vi "File IO.vi"() -> ()   [LabVIEW 2018]
uses:
  <vilib>/Utility/sysdir.llb/System Directory Type.ctl
  <vilib>/Utility/file.llb/Write Delimited Spreadsheet (DBL).vi
  <vilib>/Utility/file.llb/Write Delimited Spreadsheet (string).vi
panel:
  out "Waveform Chart":dbl[](graph)
  in  "Disabled":T1(ring)
  in  "Slide 2":dbl(slide) scale=-100.0..100.0
  in  "Slide":dbl(slide) scale=-100.0..100.0
  in  "Boolean":bool
  in  "Send":bool
  in  "stop":bool
  in  "Cluster":T2
  in  "count":i32
  out "error out 3":errorcluster
  out "text 2":string
  out "error out 2":errorcluster
  in  "text":string
  out "error out":errorcluster
  out "appended path":path
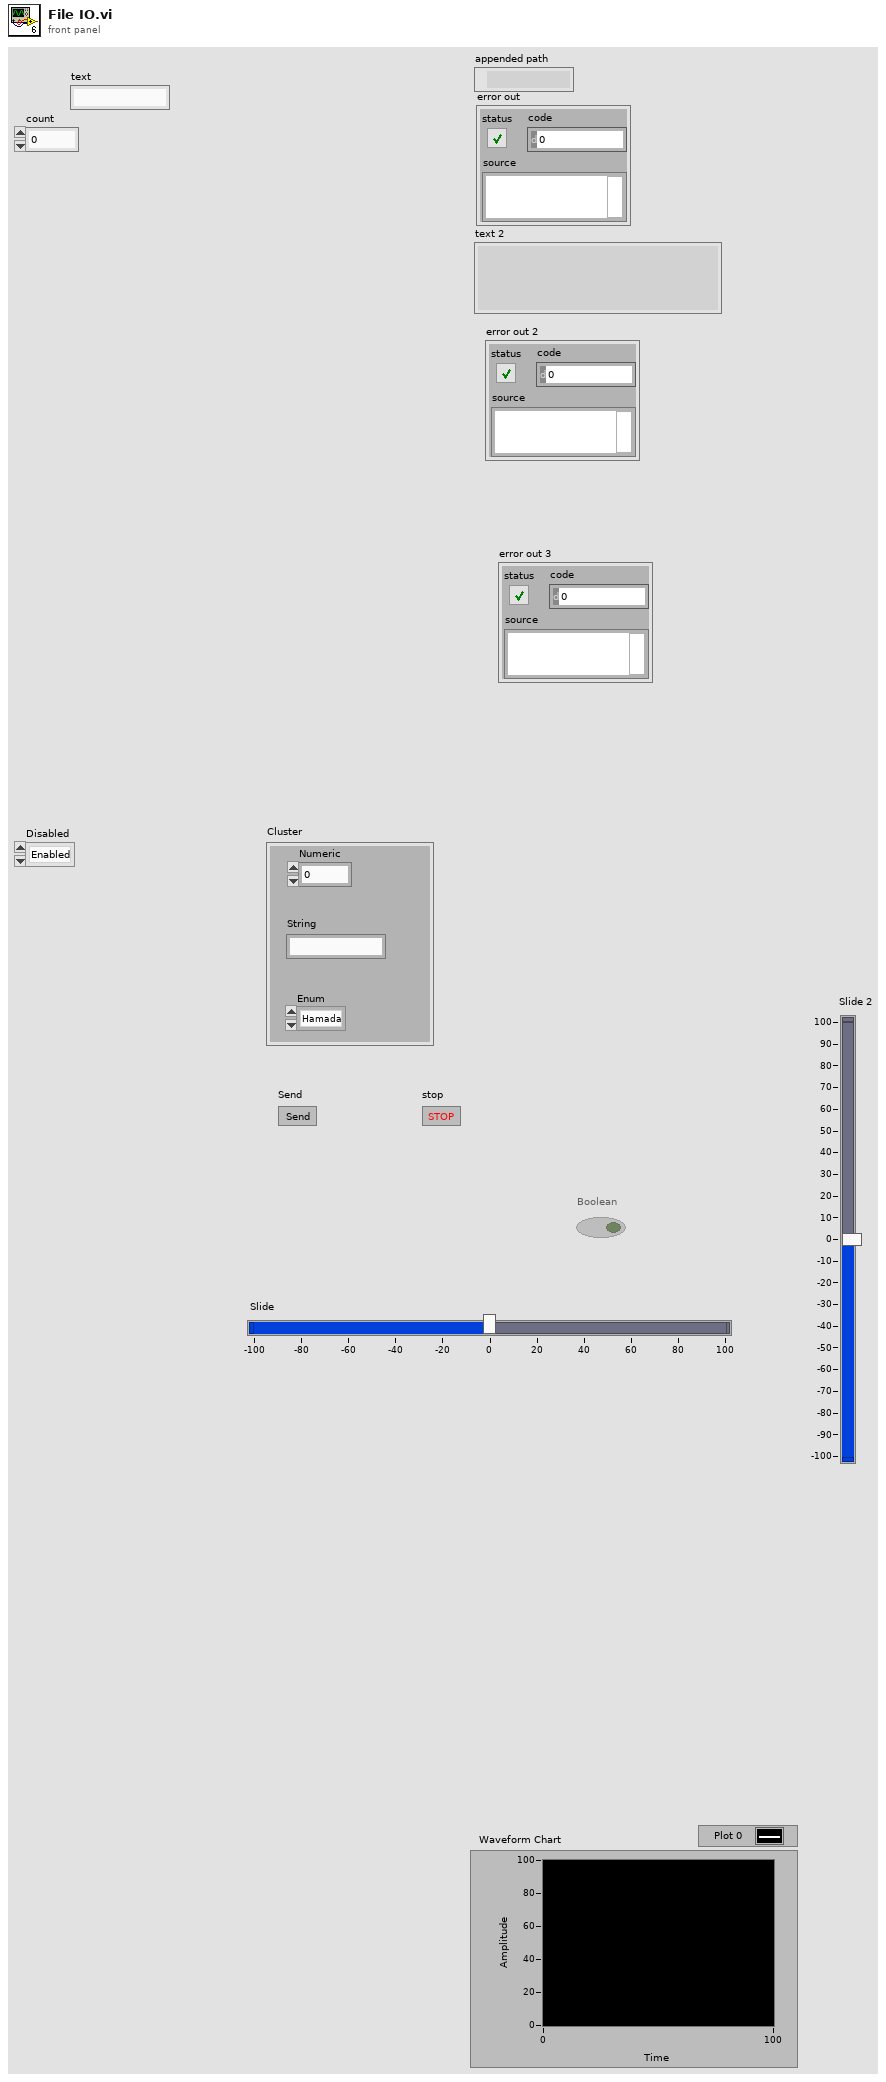
[diagram p1: front panel]
types:
  T1 = enum8{"Enabled", "Disabled", "Disabled and Grayed Out"}
  T2 = cluster{"Numeric":dbl, "String":string, "Enum":enum16{"Hamada"}}
  T3 = typedef "System Directory Type.ctl" = i32
  T4 = enum16{"open", "replace", "create", "open or create", "replace or create", "replace or create with confirmation"}
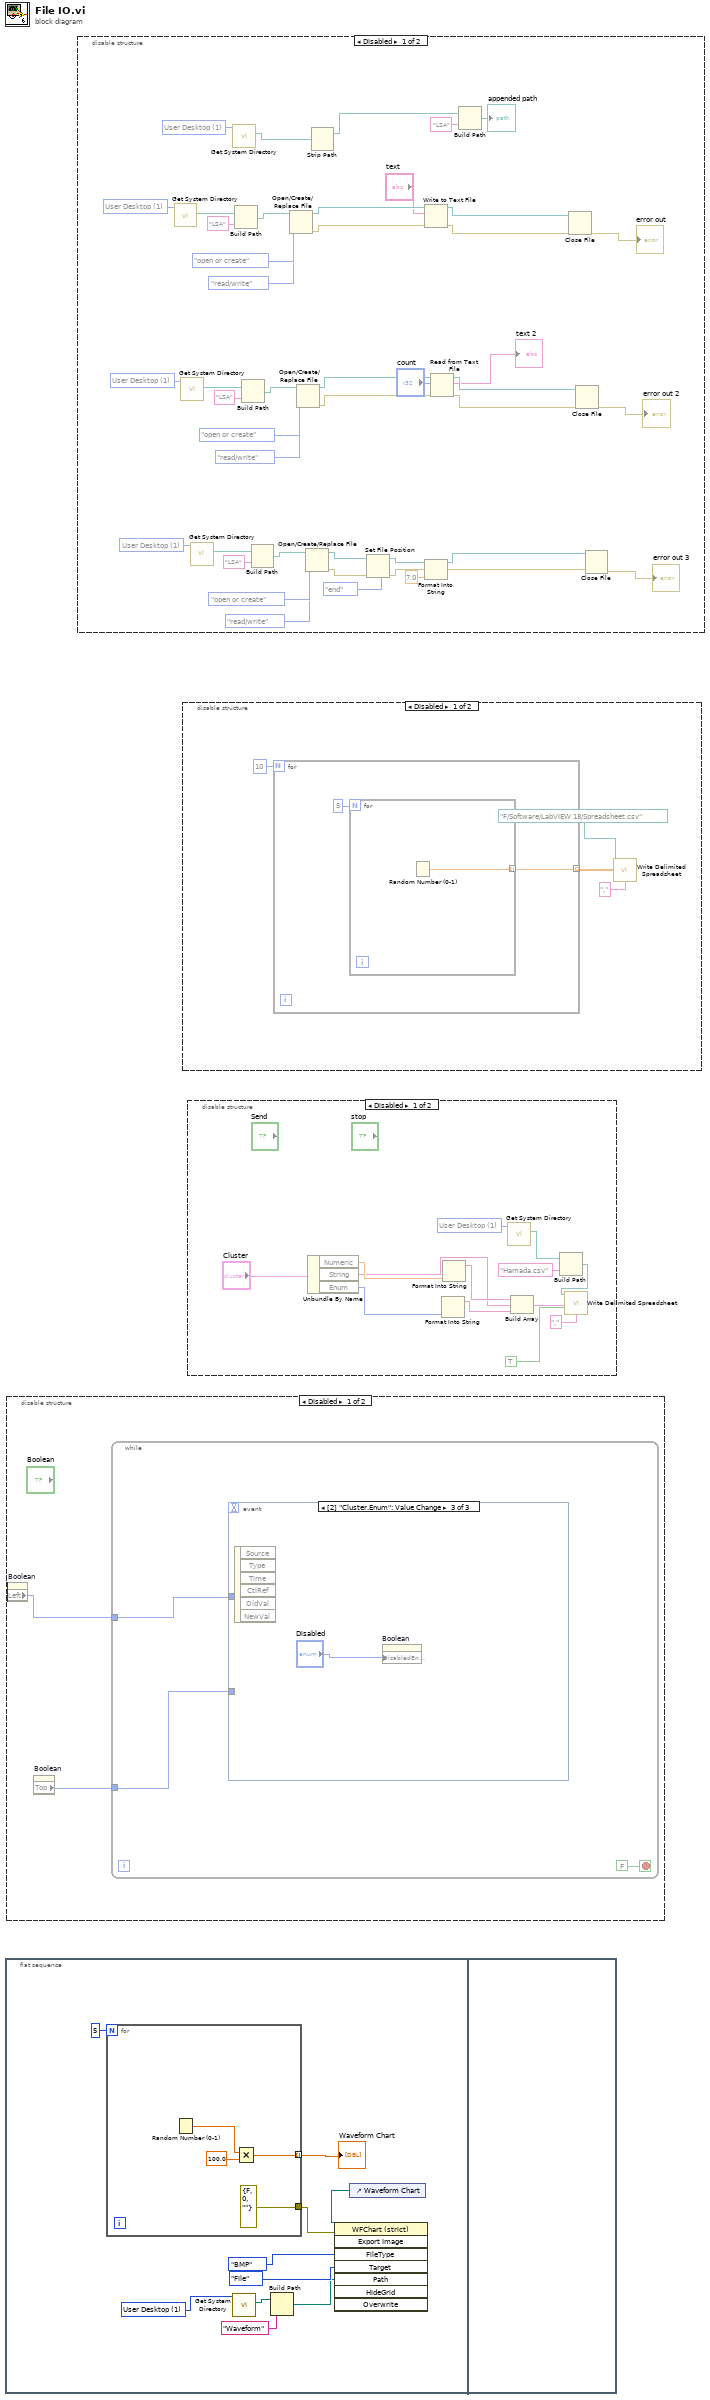
[diagram p0: block diagram]
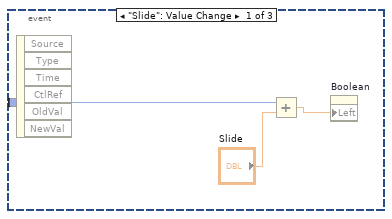
[diagram p2: hidden frame]
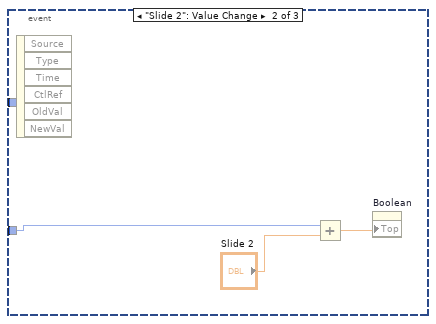
[diagram p3: hidden frame]
diagram:
  n1 = flat-sequence {
    frame #0 {
      w2 = T3 1 items=["User Home"=0, "User Desktop"=1, "User Documents"=2, "User Application Data"=3, "User Preferences"=4, "User Temporary"=5, "Public Documents"=6, "Public Application Data"=7, "Public Preferences"=8, "Public Cache"=13, "System Core Libraries"=9, "System Installed Libraries"=10, "Application Files"=11, "Boot Volume Root"=12] ("system directory type")
      n2 = for {
        N: 5 -> [_]
        tunnel: [w12] -> w9 mode=indexing
        tunnel: [errorcluster {"status"=FALSE, "code"=0, "source"=""} ("error in (no error)")] -> w7
        n3 = Random Number (0-1)() -> (number: 0 to 1=w14:dbl)
        n4 = Multiply(x=w14, y=100.0) -> (x*y=w12:dbl)
      }
      "Waveform Chart" <- w9
      n5 = call <vilib>:"Get System Directory.vi"("system directory type"=w2) -> ("system directory"=w3:path)  [unwired: 10 in]
      n6 = Build Path(base path=w3, name or relative path="Waveform") -> (appended path=w1:path)
      n7 = control-ref of="Waveform Chart"() -> (w8:refnum<vi>)
      n8 = invoke class="WFChart (strict)" method="Export Image"(reference=w8, error in=w7, "FileType"=enum32{"BMP", "EPS", "EMF", "PICT"}."BMP" ("File Type"), "Target"=enum32{"File", "Clipboard"}."File", "Path"=w1) -> ()  [unwired: 3 in, 8 out]
    }
    frame #1 {
    }
  }
  n9 = disable-structure shown="Disabled" {
    frame Disabled {
      n10 = property on="Boolean" class="Bool (strict)"() -> ("Left"=w16:i32)  [unwired: 2 in, 2 out]
      n11 = property on="Boolean" class="Bool (strict)"() -> ("Top"=w15:i32)  [unwired: 2 in, 2 out]
      n12 = while {
        tunnel: w16 -> [w19]
        tunnel: w15 -> [w17]
        stop <- FALSE stop-if-true
        n13 = event shown="[2] \"Cluster.Enum\": Value Change" {
          selector: _ -> [_ _ _]
          dyn-events: _ -> [_ _ _]
          timeout: _ -> [_ _ _]
          tunnel: w19 -> [w22 _ _]
          tunnel: w17 -> [_ w24 _]
          event "Slide": Value Change {
            n14 = event-data() -> ()  [unwired: 1 in, 6 out]
            n15 = Add(x=w22, y="Slide") -> (x+y=w20:dbl)
            n16 = property on="Boolean" class="Bool (strict)"("Left"=w20) -> ()  [unwired: 2 in, 2 out]
          }
          event "Slide 2": Value Change {
            n17 = event-data() -> ()  [unwired: 1 in, 6 out]
            n18 = Add(x=w24, y="Slide 2") -> (x+y=w23:dbl)
            n19 = property on="Boolean" class="Bool (strict)"("Top"=w23) -> ()  [unwired: 2 in, 2 out]
          }
          event "Cluster.Enum": Value Change {
            n20 = event-data() -> ()  [unwired: 1 in, 6 out]
            n21 = property on="Boolean" class="Bool (strict)"("DisabledEnum"="Disabled") -> ()  [unwired: 2 in, 2 out]
          }
        }
      }
    }
    frame Enabled {
    }
  }
  n22 = disable-structure shown="Disabled" {
    frame Disabled {
      w39 = T3 1 items=["User Home"=0, "User Desktop"=1, "User Documents"=2, "User Application Data"=3, "User Preferences"=4, "User Temporary"=5, "Public Documents"=6, "Public Application Data"=7, "Public Preferences"=8, "Public Cache"=13, "System Core Libraries"=9, "System Installed Libraries"=10, "Application Files"=11, "Boot Volume Root"=12] ("system directory type")
      w51 = T3 1 items=["User Home"=0, "User Desktop"=1, "User Documents"=2, "User Application Data"=3, "User Preferences"=4, "User Temporary"=5, "Public Documents"=6, "Public Application Data"=7, "Public Preferences"=8, "Public Cache"=13, "System Core Libraries"=9, "System Installed Libraries"=10, "Application Files"=11, "Boot Volume Root"=12] ("system directory type")
      w58 = T3 1 items=["User Home"=0, "User Desktop"=1, "User Documents"=2, "User Application Data"=3, "User Preferences"=4, "User Temporary"=5, "Public Documents"=6, "Public Application Data"=7, "Public Preferences"=8, "Public Cache"=13, "System Core Libraries"=9, "System Installed Libraries"=10, "Application Files"=11, "Boot Volume Root"=12] ("system directory type")
      w60 = T3 1 items=["User Home"=0, "User Desktop"=1, "User Documents"=2, "User Application Data"=3, "User Preferences"=4, "User Temporary"=5, "Public Documents"=6, "Public Application Data"=7, "Public Preferences"=8, "Public Cache"=13, "System Core Libraries"=9, "System Installed Libraries"=10, "Application Files"=11, "Boot Volume Root"=12] ("system directory type")
      n23 = call <vilib>:"Get System Directory.vi"("system directory type"=w58) -> ("system directory"=w57:path)  [unwired: 10 in]
      n24 = call <vilib>:"Get System Directory.vi"("system directory type"=w51) -> ("system directory"=w52:path)  [unwired: 10 in]
      n25 = call <vilib>:"Get System Directory.vi"("system directory type"=w39) -> ("system directory"=w38:path)  [unwired: 10 in]
      n26 = call <vilib>:"Get System Directory.vi"("system directory type"=w60) -> ("system directory"=w61:path)  [unwired: 10 in]
      n27 = Build Path(base path=w57, name or relative path="LSA") -> (appended path=w56:path)
      n28 = Build Path(base path=w52, name or relative path="LSA") -> (appended path=w53:path)
      n29 = Build Path(base path=w38, name or relative path="LSA") -> (appended path=w37:path)
      n30 = Open/Create/Replace File(file path (use dialog)=w56, operation (0:open)=T4."open or create", access (0:read/write)=enum16{"read/write", "read-only", "write-only"}."read/write") -> (refnum out=w68:refnum<file>, error out=w64:errorcluster)  [unwired: 3 in, 1 out]
      n31 = Open/Create/Replace File(file path (use dialog)=w53, operation (0:open)=T4."open or create", access (0:read/write)=enum16{"read/write", "read-only", "write-only"}."read/write") -> (refnum out=w47:refnum<file>, error out=w46:errorcluster)  [unwired: 3 in, 1 out]
      n32 = Open/Create/Replace File(file path (use dialog)=w37, operation (0:open)=T4."open or create", access (0:read/write)=enum16{"read/write", "read-only", "write-only"}."read/write") -> (refnum out=w30:refnum<file>, error out=w29:errorcluster)  [unwired: 3 in, 1 out]
      n33 = Strip Path(path=w61) -> (stripped path=w71:path)  [unwired: 1 out]
      n34 = Set File Position(refnum=w30, from (0:start)=enum16{"start", "end", "current"}."end", error in=w29) -> (refnum out=w31:refnum<file>, error out=w32:errorcluster)  [unwired: 1 in]
      n35 = Write to Text File(file (use dialog)=w68, text="text", error in=w64) -> (refnum out=w67:refnum<file>, error out=w63:errorcluster)  [unwired: 1 in, 1 out]
      n36 = Format Into String(initial string=w31, error in=w32, 7.0 ("input 1")) -> (resulting string=w35:refnum<file>, error out=w33:errorcluster)  [unwired: 1 in]
      n37 = Read from Text File(file (use dialog)=w47, count="count", error in=w46) -> (refnum out=w44:refnum<file>, text=→"text 2":string, error out=w45:errorcluster)  [unwired: 1 in, 1 out]
      n38 = Build Path(base path=w71, name or relative path="LSA") -> (appended path=→"appended path":path)
      n39 = Close File(refnum=w67, error in=w63) -> (error out=→"error out":errorcluster)  [unwired: 1 out]
      n40 = Close File(refnum=w44, error in=w45) -> (error out=→"error out 2":errorcluster)  [unwired: 1 out]
      n41 = Close File(refnum=w35, error in=w33) -> (error out=→"error out 3":errorcluster)  [unwired: 1 out]
    }
    frame Enabled {
    }
  }
  n42 = disable-structure shown="Disabled" {
    frame Disabled {
      n43 = for {
        N: 10 -> [_]
        tunnel: [w77] -> w74 mode=indexing
        n44 = for {
          N: 5 -> [_]
          tunnel: [w78] -> w77 mode=indexing
          n45 = Random Number (0-1)() -> (number: 0 to 1=w78:dbl)
        }
      }
      n46 = call-poly <vilib>:"Write Delimited Spreadsheet.vi"("file path (dialog if empty)"=path "F:/Software/LabVIEW 18/Spreadsheet.csv", "2D data"=w74, "delimiter (\\t)"="," ("delimiter (\\t)")) -> ()  [unwired: 11 in, 2 out]
    }
    frame Enabled {
    }
  }
  n47 = disable-structure shown="Disabled" {
    frame Disabled {
      w84 = T3 1 items=["User Home"=0, "User Desktop"=1, "User Documents"=2, "User Application Data"=3, "User Preferences"=4, "User Temporary"=5, "Public Documents"=6, "Public Application Data"=7, "Public Preferences"=8, "Public Cache"=13, "System Core Libraries"=9, "System Installed Libraries"=10, "Application Files"=11, "Boot Volume Root"=12] ("system directory type")
      n48 = Unbundle By Name("Cluster") -> ("Numeric"=w90:dbl, "String"=w87:string, "Enum"=w89:enum16{"Hamada"})
      n49 = Format Into String(w89) -> (resulting string=w86:string)  [unwired: 3 in, 1 out]
      n50 = Format Into String(w90) -> (resulting string=w88:string)  [unwired: 3 in, 1 out]
      n51 = call <vilib>:"Get System Directory.vi"("system directory type"=w84) -> ("system directory"=w82:path)  [unwired: 10 in]
      n52 = Build Array(w88, w87, w86) -> (w85:string[])
      n53 = Build Path(base path=w82, name or relative path="Hamada.csv") -> (appended path=w80:path)
      n54 = call-poly <vilib>:"Write Delimited Spreadsheet.vi"("file path (dialog if empty)"=w80, "1D data"=w85, "append to file? (new file:F)"=TRUE, "delimiter (\\t)"="," ("delimiter (\\t)")) -> ()  [unwired: 10 in, 2 out]
    }
    frame Enabled {
    }
  }
